vi "Create particle pathline.vi"(2 "Colour":T1={"Red"=1.0, "Green"=1.0, "Blue"=1.0, "Alpha"=1.0}, 3 "Render mode":T2(ring)=enum."Wireframe", 4 "Points":sgl[][](array[numeric])) -> (0 "Error out":errorcluster, 1 "Pathline out":refnum<vi>)   [LabVIEW 2017]
uses:
  <vilib>/Utility/miscctls.llb/LVRGBAColorTypeDef.ctl
  <vilib>/picture/3D Picture Control/Object/Create Object (drawable).vi
  <vilib>/Utility/miscctls.llb/LV3DPointTypeDef.ctl
  <vilib>/picture/3D Picture Control/NI_3D Picture Control.lvlib
panel:
  # "PN 23/10/17"
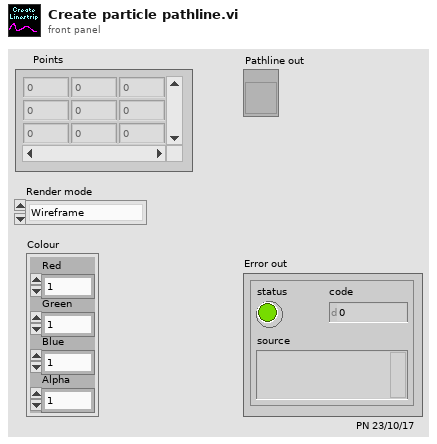
[diagram p1: front panel]
types:
  T1 = typedef "LVRGBAColorTypeDef.ctl" = cluster{"Red":sgl, "Green":sgl, "Blue":sgl, "Alpha":sgl}
  T2 = enum16{"Inherit Value", "Points", "Wireframe", "Polygons"}
  T3 = enum16{"Inherit Material", "Use entire Material", "Ignore Ambient", "Ignore Diffuse", "Ignore Specular", "Ignore Emission", "Ignore Ambient and Diffuse"}
  T4 = enum16{"Overall", "Per Primitive", "Per Vertex", "Binding Off"}
  T5 = enum16{"Points", "Lines", "Line Strip", "Line Loop", "Triangles", "Triangle Strip", "Triangle Fan", "Quads", "Quad Strip", "Polygon"}
  T6 = enum16{"Inherit Value", "No Culling", "Cull Back Face", "Cull Front Face", "Cull Both Faces"}
  T7 = enum16{"Inherit Value", "Counterclockwise", "Clockwise"}
  T8 = typedef "LV3DPointTypeDef.ctl" = cluster{"X":sgl, "Y":sgl, "Z":sgl}
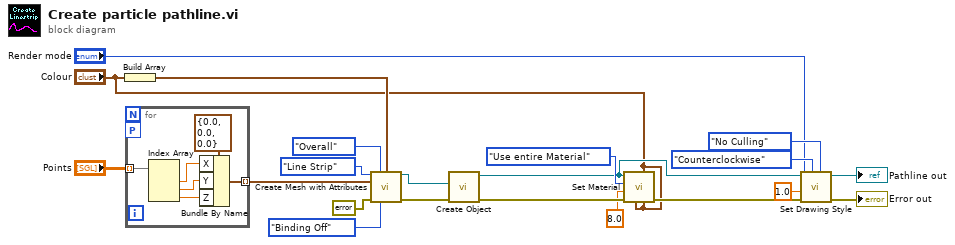
[diagram p0: block diagram]
diagram:
  n1 = Build Array("Colour") -> (w3:T1[])
  n2 = for {
    tunnel: [w23] -> w13 mode=indexing
    tunnel: "Points" -> [w27] mode=indexing
    workers-P: _ -> [_]
    n3 = Index Array(array=w27) -> (element #1=w26:sgl, element #2=w25:sgl, element #3=w24:sgl)  [unwired: 3 in]
    n4 = Bundle By Name(cluster=T8 {"X"=0.0, "Y"=0.0, "Z"=0.0} ("3D Point"), "X"=w26, "Y"=w25, "Z"=w24) -> (w23:T8)
  }
  n5 = call <vilib>:"Create Mesh with Attributes.vi"("Draw Mode"=T5."Line Strip", "Color Binding Mode"=T4."Overall", "Color Array"=w3, "Vertex Array"=w13, "error in (no error)"=errorcluster {"status"=FALSE, "code"=0, "source"=""}, "Normal Binding Mode"=T4."Binding Off") -> ("New Mesh Refnum"=w15:refnum<vi>, "error out"=w16:errorcluster)  [unwired: 8 in]
  n6 = call-poly <vilib>:"Create Object.vi"("error in (no error)"=w16, "Geometry"=w15) -> ("error out"=w8:errorcluster, "Scene:New Object"=w4:refnum<vi>)  [unwired: 8 in]
  n7 = call <vilib>:"Set Material.vi"("Diffuse"="Colour", "Specular"="Colour", "Emission"="Colour", "error in (no error)"=w8, "Shininess"=sgl 8.0, "Color Mode"=T3."Use entire Material", "Scene Object In"=w4) -> ("error out"=w7:errorcluster)  [unwired: 3 in, 1 out]
  n8 = call <vilib>:"Set Drawing Style.vi"("Face Culling Mode"=T6."No Culling", "Frontface Mode"=T7."Counterclockwise", "error in (no error)"=w7, "Size"=1.0, "Mode"="Render mode", "Scene Object In"=w4) -> ("error out"=→"Error out":errorcluster, "Scene Object Out"=→"Pathline out":refnum<vi>)  [unwired: 4 in]
